vi "UnknownAction.vi"(5 "Data":variant, 6 "MergeErrors":bool caption="MergeErrors (F)", 7 "Object":refnum<class "TAFBaseGUI.lvclass">, 8 "ErrorIn":errorcluster, 9 "Parameters":string, 10 "SubCommand":string, 11 "FullCommand":string) -> (0 "ErrorOut":errorcluster)   [LabVIEW 2021, in "TAFBaseGUI.lvclass"]
uses:
  TAFBaseGUI.lvclass
  TAFBaseGUI.lvclass/TAFBaseGUI.ctl
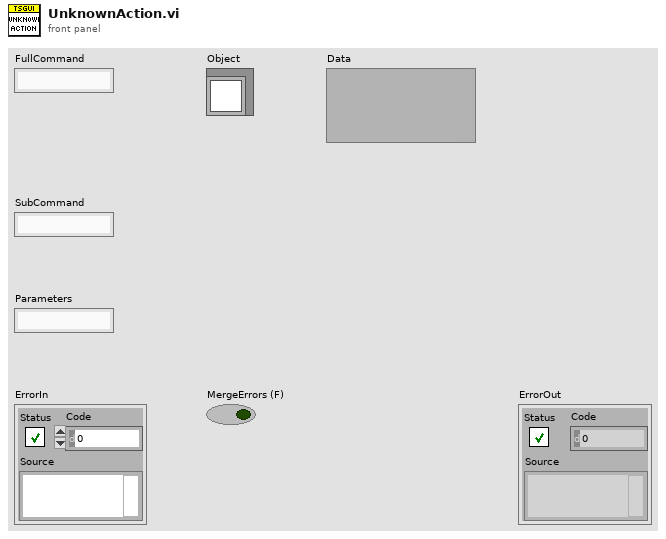
[diagram p1: front panel]
types:
  T1 = cluster{"Name":string, "FullCommand":string, "SubCommand":string, "Parameters":string, "Data":variant}
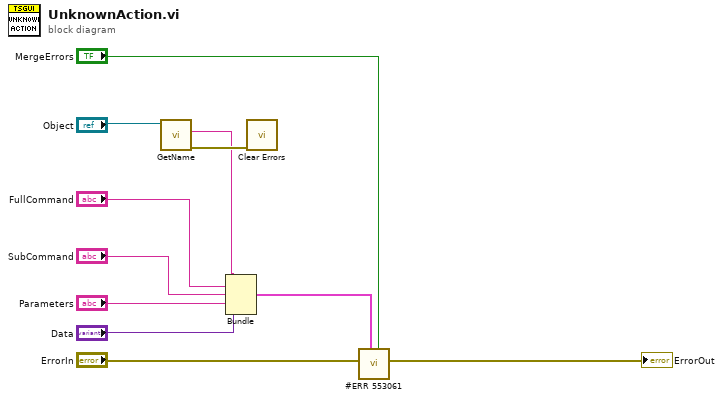
[diagram p0: block diagram]
diagram:
  n1 = call-dynamic "GetName.vi"("reference in"="Object") -> ("error out"=w9:errorcluster, "Name"=w1:string)  [unwired: 8 in, 1 out]
  n2 = Bundle("Name"=w1, "FullCommand"="FullCommand", "SubCommand"="SubCommand", "Parameters"="Parameters", "Data"="Data") -> (w3:T1)  [unwired: 1 in]
  n3 = call <vilib>:"Clear Errors.vi"("error in (no error)"=w9) -> ()  [unwired: 5 in, 2 out]
  n4 = call "#ERR 553061"("MergeErrors"="MergeErrors", "Data"=w3, "error in (no error)"="ErrorIn") -> ("error out"=→"ErrorOut":errorcluster)  [unwired: 8 in]
